vi "Writer-Reader.vi"() -> ()   [LabVIEW 2019]
doc: "Demonstrates using the Writer and Reader VIs to explicitly encode and decode LabVIEW types and values. This is more verbose, but it can be more performant and minimize memory allocations."
uses:
  vi.lib/Field R&D Services/LabPack/Public/Writer/Writer.lvclass/Writer.ctl
  vi.lib/Field R&D Services/LabPack/Public/Reader/Reader.lvclass/Reader.ctl
  vi.lib/Field R&D Services/LabPack/Public/Writer/Private/Handle Error.vi
  vi.lib/Field R&D Services/LabPack/Public/Reader/Public/Raw/Read Bytes.vi
  vi.lib/Field R&D Services/LabPack/Public/Reader/Private/Read Bytes by Value.vi
  vi.lib/Field R&D Services/LabPack/Public/Reader/Private/Handle Error.vi
  vi.lib/Field R&D Services/LabPack/Public/Writer/Public/Status/Read Is Error.vi
  vi.lib/Field R&D Services/LabPack/Public/Writer/Public/Status/Read Status.vi
  vi.lib/Field R&D Services/LabPack/Public/Writer/Public/Status/Read Status Message.vi
  vi.lib/Field R&D Services/LabPack/Public/Reader/Public/Status/Read Status.vi
  vi.lib/Field R&D Services/LabPack/Public/Reader/Public/Status/Read Status Message.vi
  vi.lib/Field R&D Services/LabPack/Public/Reader/Public/Status/Read Is Error.vi
  vi.lib/Field R&D Services/LabPack/Public/Writer/Private/Begin by Value.vi
  vi.lib/Field R&D Services/LabPack/Public/Writer/Private/Begin Map by Value.vi
  vi.lib/Field R&D Services/LabPack/Public/Utility/Status Code.vi
  <vilib>/Utility/error.llb/Error Cluster From Error Code.vi
  vi.lib/Field R&D Services/LabPack/Public/Writer/Private/End Map by Value.vi
  vi.lib/Field R&D Services/LabPack/Public/Writer/Private/End by Value.vi
  vi.lib/Field R&D Services/LabPack/Public/Reader/Private/Begin by Value.vi
  vi.lib/Field R&D Services/LabPack/Public/Reader/Private/Begin Map by Value.vi
  vi.lib/Field R&D Services/LabPack/Public/Reader/Public/String/Begin Str.vi
  vi.lib/Field R&D Services/LabPack/Public/Reader/Private/Begin Str by Value.vi
  vi.lib/Field R&D Services/LabPack/Public/Reader/Public/String/End Str.vi
  vi.lib/Field R&D Services/LabPack/Public/Reader/Private/End Str by Value.vi
  vi.lib/Field R&D Services/LabPack/Public/Reader/Private/End Map by Value.vi
  vi.lib/Field R&D Services/LabPack/Public/Reader/Private/End by Value.vi
  vi.lib/Field R&D Services/LabPack/Public/Writer/Writer.lvclass
  vi.lib/Field R&D Services/LabPack/Public/Reader/Reader.lvclass
panel:
  out "Value 2":u32
  out "Key 2":string
  out "Value 1":bool
  out "Key 1":string
  out "Map Count":u32
  out "Encoded Data":string
  # "Run the VI to see LabVIEW types encoded as MessagePack data using the Writer class API and then decoded using the Reader class API"
  # "Decoded Data"
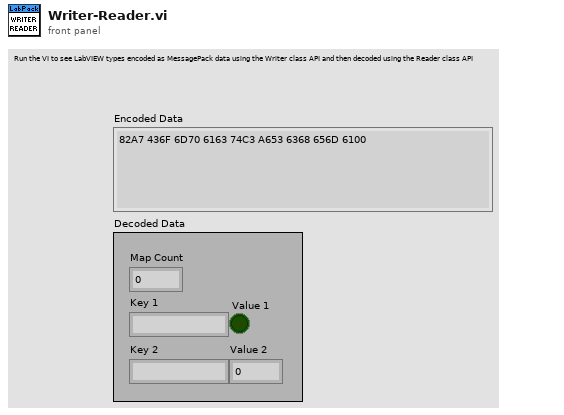
[diagram p1: front panel]
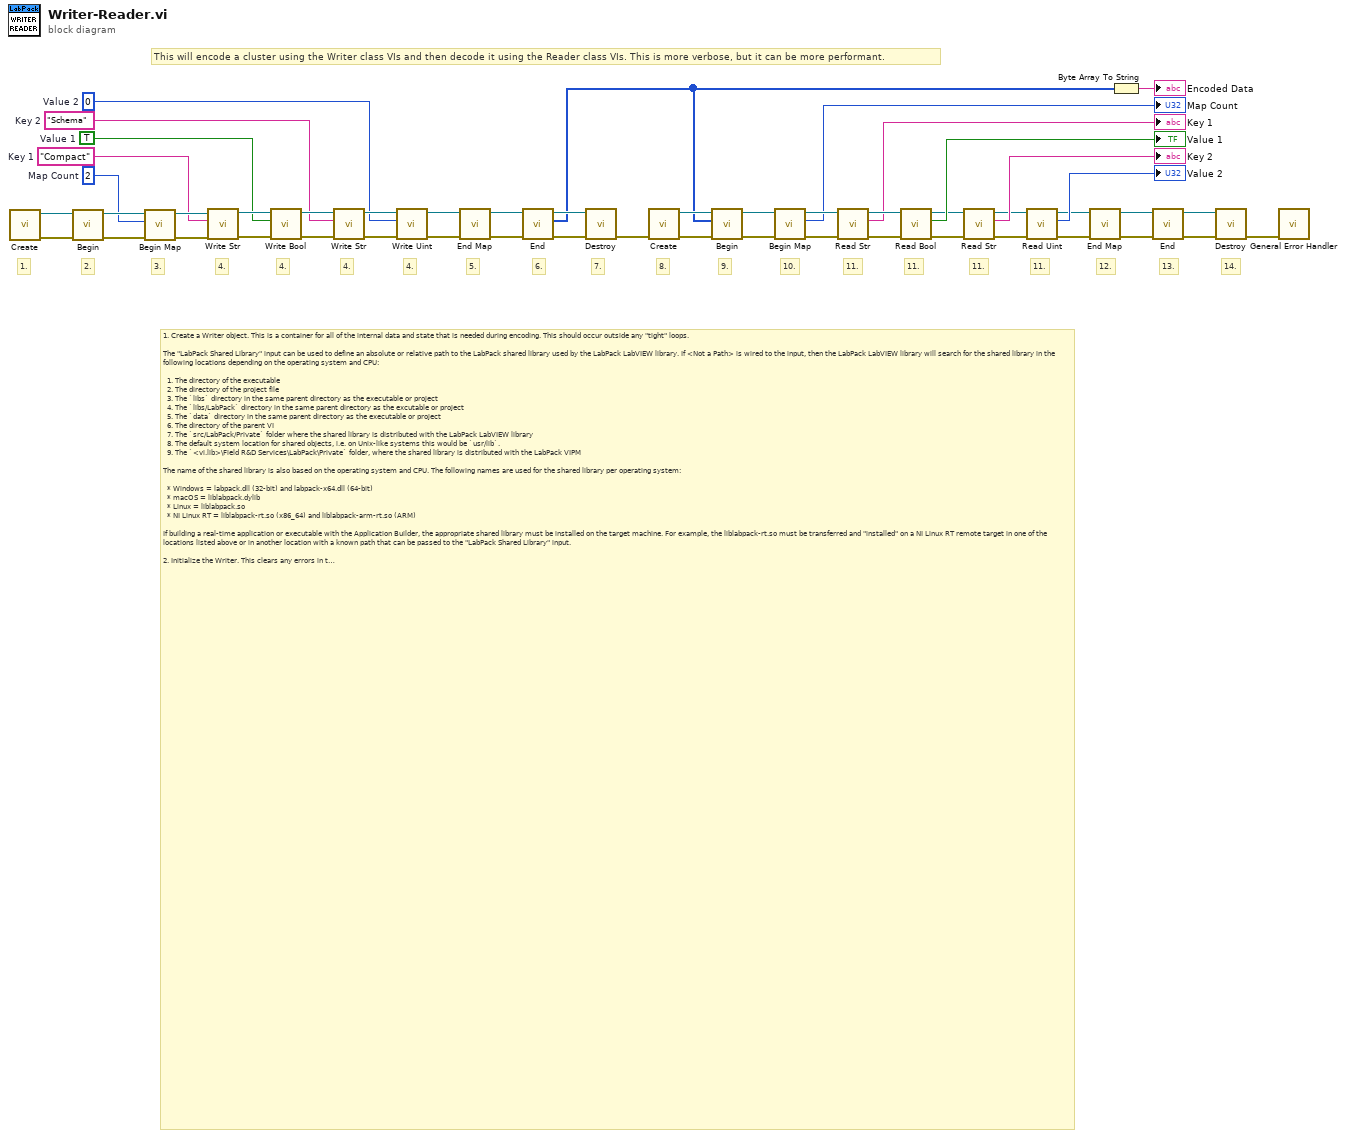
[diagram p0: block diagram]
diagram:
  w33 = u64 0  # Value 2
  w36 = "Schema"  # Key 2
  w39 = TRUE  # Value 1
  w42 = "Compact"  # Key 1
  w45 = u32 2  # Map Count
  # "14."
  # "13."
  # "12."
  # "11."
  # "11."
  # "11."
  # "11."
  # "10."
  # "9."
  # "8."
  # "7."
  # "6."
  # "5."
  # "4."
  # "4."
  # "4."
  # "4."
  # "3."
  # "2."
  # "1."
  # "This will encode a cluster using the Writer class VIs and then decode it using the Reader class VIs. This is more verbose, but it can be more performant."
  # "1. Create a Writer object. This is a container for all of the internal data and state that is needed during encoding. This should occur outside any \"tight\" loops.\n\nThe \"LabPack Shared Library\" input can be used to define an absolute or relative path to the LabPack shared library used by the LabPack LabVIEW library. If <Not a Path> is wired to the input, then the LabPack LabVIEW library will search for the shared library in the following locations depending on the operating system and CPU: \n\n  1. The directory of the executable \n  2. The directory of the project file\n  3. The `libs` directory in the same parent directory as the executable or project\n  4. The `libs/LabPack` directory in the same parent directory as the excutable or project\n  5. The `data` directory in the same parent directory as the executable or project\n  6. The directory of the parent VI\n  7. The `src/LabPack/Private` folder where the shared library is distributed with the LabPack LabVIEW library\n  8. The default system location for shared objects, i.e. on Unix-like systems this would be `usr/lib`.\n  9. The `<vi.lib>\\Field R&D Services\\LabPack\\Private` folder, where the shared library is distributed with the LabPack VIPM\n\nThe name of the shared library is also based on the operating system and CPU. The following names are used for the shared library per operating system:\n\n  * Windows = labpack.dll (32-bit) and labpack-x64.dll (64-bit)\n  * macOS = liblabpack.dylib\n  * Linux = liblabpack.so\n  * NI Linux RT = liblabpack-rt.so (x86_64) and liblabpack-arm-rt.so (ARM)\n\nIf building a real-time application or executable with the Application Builder, the appropriate shared library must be installed on the target machine. For example, the liblabpack-rt.so must be transferred and \"installed\" on a NI Linux RT remote target in one of the locations listed above or in another location with a known path that can be passed to the \"LabPack Shared Library\" input.\n\n2. Initialize the Writer. This clears any errors in the decoder and allocates memory. This allows the Writer object to be created once and reuses without having to destroy the Writer object.\n\n3. Create a map with a specified number of elements. A map is an array of key-value pairs.\n\n4. Write the key-value pairs for the map. These can be safely executed inside a \"tight\" loop. Note, the keys do not need to be strings, but typically strings are used as keys.\n\n5. Finish encoding the map. This must be called after all of the key-value pairs, or elements, have been encoded.\n\n6. Finish the encoding and obtain the binary MessagePack data. After this is called, the Begin VI can be used to resuse the Writer object without destroying the Writer object.\n\n7. Destroy the Writer object because it is no longer used and this may free up resources.\n\n8. Create a Reader object. This is a container for all of the internal data and state that is needed during decoding. This should occur outside any \"tight\" loops.\n\n9. Initialize the Reader with the encoded binary MessagePack data. This will allocate memory. This also clears any errors and allows the Reader object to be reused.\n\n10. Read a map and get the number of elements (key-value pairs). A map is expected, but if the MessagePack object is NOT a map, an error will occurr.\n\n11. Read the key-value pairs of the map. Strings are expected for the keys, a boolean is expected for the first value, and an integer is expected for second value. An error occurs if the MessagePack objects are not as expected.\n\n12. Finish decoding the map. This must be called after all of the key-value pairs, or elements, have been decoded.\n\n13. Finish decoding. This must be called after decoding all of the MessagePack data. After this is called, the Begin VI can be called to reuse the Reader object without detsroying the object.\n\n14. Destroy the Reader object because it is no longer used and this may free up resources."
  n1 = call "Create.vi"() -> ("Error Out"=w48:errorcluster, "Writer"=w49:refnum<class "Writer.lvclass">)  [unwired: 10 in]
  n2 = call-poly "Begin.vi"("Error In"=w48, "Writer In"=w49) -> ("Error Out"=w46:errorcluster, "Writer Out"=w47:refnum<class "Writer.lvclass">)  [unwired: 8 in]
  n3 = call-poly "Begin Map.vi"("Error In"=w46, "Elements Count"=w45, "Writer In"=w47) -> ("Error Out"=w43:errorcluster, "Writer Out"=w44:refnum<class "Writer.lvclass">)  [unwired: 7 in]
  n4 = call "Write Str.vi"("Error In"=w43, "Value"=w42, "Writer In"=w44) -> ("Error Out"=w40:errorcluster, "Writer Out"=w41:refnum<class "Writer.lvclass">)  [unwired: 7 in]
  n5 = call "Write Bool.vi"("Error In"=w40, "Value"=w39, "Writer In"=w41) -> ("Error Out"=w37:errorcluster, "Writer Out"=w38:refnum<class "Writer.lvclass">)  [unwired: 7 in]
  n6 = call "Write Str.vi"("Error In"=w37, "Value"=w36, "Writer In"=w38) -> ("Error Out"=w34:errorcluster, "Writer Out"=w35:refnum<class "Writer.lvclass">)  [unwired: 7 in]
  n7 = call "Write Uint.vi"("Error In"=w34, "Value"=w33, "Writer In"=w35) -> ("Error Out"=w31:errorcluster, "Writer Out"=w32:refnum<class "Writer.lvclass">)  [unwired: 7 in]
  n8 = call-poly "End Map.vi"("Error In"=w31, "Writer In"=w32) -> ("Error Out"=w29:errorcluster, "Writer Out"=w30:refnum<class "Writer.lvclass">)  [unwired: 8 in]
  n9 = call-poly "End.vi"("Error In"=w29, "Writer In"=w30) -> ("Error Out"=w27:errorcluster, "Data"=w23:u8[], "Writer Out"=w28:refnum<class "Writer.lvclass">)  [unwired: 7 in]
  n10 = call "Destroy.vi"("Error In"=w27, "Writer"=w28) -> ("Error Out"=w26:errorcluster)  [unwired: 9 in]
  n11 = call "Create.vi"("Error In"=w26) -> ("Error Out"=w24:errorcluster, "Reader"=w25:refnum<class "Reader.lvclass">)  [unwired: 9 in]
  n12 = call-poly "Begin.vi"("Error In"=w24, "Msgpack Data"=w23, "Reader In"=w25) -> ("Error Out"=w21:errorcluster, "Reader Out"=w22:refnum<class "Reader.lvclass">)  [unwired: 7 in]
  n13 = call-poly "Begin Map.vi"("Error In"=w21, "Reader In"=w22) -> ("Error Out"=w19:errorcluster, "Count"=→"Map Count":u32, "Reader Out"=w20:refnum<class "Reader.lvclass">)  [unwired: 7 in]
  n14 = call "Read Str.vi"("Error In"=w19, "Reader In"=w20) -> ("Error Out"=w16:errorcluster, "Value"=→"Key 1":string, "Reader Out"=w17:refnum<class "Reader.lvclass">)  [unwired: 7 in]
  n15 = call "Read Bool.vi"("Error In"=w16, "Reader In"=w17) -> ("Error Out"=w12:errorcluster, "Value"=→"Value 1":bool, "Reader Out"=w13:refnum<class "Reader.lvclass">)  [unwired: 7 in]
  n16 = call "Read Str.vi"("Error In"=w12, "Reader In"=w13) -> ("Error Out"=w9:errorcluster, "Value"=→"Key 2":string, "Reader Out"=w10:refnum<class "Reader.lvclass">)  [unwired: 7 in]
  n17 = call "Read Uint.vi"("Error In"=w9, "Reader In"=w10) -> ("Error Out"=w6:errorcluster, "Value"=→"Value 2":u32, "Reader Out"=w7:refnum<class "Reader.lvclass">)  [unwired: 7 in]
  n18 = call-poly "End Map.vi"("Error In"=w6, "Reader In"=w7) -> ("Error Out"=w4:errorcluster, "Reader Out"=w5:refnum<class "Reader.lvclass">)  [unwired: 8 in]
  n19 = Byte Array To String(unsigned byte array=w23) -> (string=→"Encoded Data":string)
  n20 = call-poly "End.vi"("Error In"=w4, "Reader In"=w5) -> ("Error Out"=w2:errorcluster, "Reader Out"=w3:refnum<class "Reader.lvclass">)  [unwired: 8 in]
  n21 = call "Destroy.vi"("Error In"=w2, "Reader"=w3) -> ("Error Out"=w1:errorcluster)  [unwired: 9 in]
  n22 = call <vilib>:"General Error Handler.vi"("error in (no error)"=w1) -> ()  [unwired: 10 in, 5 out]
